vi "Get Pulse State.vi"(8 "error in (no error)":errorcluster, 11 "DAQmx Digitizer in":refnum<class "DAQmx Digitizer.lvclass">) -> (0 "error out":errorcluster, 1 "Result ready":bool, 2 "Armed":bool, 3 "DAQmx Digitizer out":refnum<class "DAQmx Digitizer.lvclass">, 4 "Recording compleste":bool)   [LabVIEW 2021, in "DAQmx Digitizer.lvclass"]
uses:
  DAQmx Digitizer.lvclass
  C:/GitHub/NHMFL_Core/Libraries/Instruments/Pulse Driver/Pulse Driver.lvclass
  Instruments/Pulse Driver/Pulse Driver.lvclass/Pulse Driver.ctl
  Instruments/Pulse Driver/Read Samples per read.vi
  Instruments/Pulse Driver/Read Samples per channel.vi
  Instruments/Pulse Driver/Read Current read position.vi
  DAQmx Digitizer.lvclass/DAQmx Digitizer.ctl
  <resource>/objmgr/daqmx.rc
panel:
  out "AvailSampPerChan 2":u32
  out "Samples per channel":i32
  out "Samples per read":i32=-1
  out "Current read position":i32
  out "AvailSampPerChan":u32
  out "RelativeTo":i32(ring)=10424 items=["First Sample"=10424, "Current Read Position"=10425, "Reference Trigger"=10426, "First Pretrigger Sample"=10427, "Most Recent Sample"=10428]
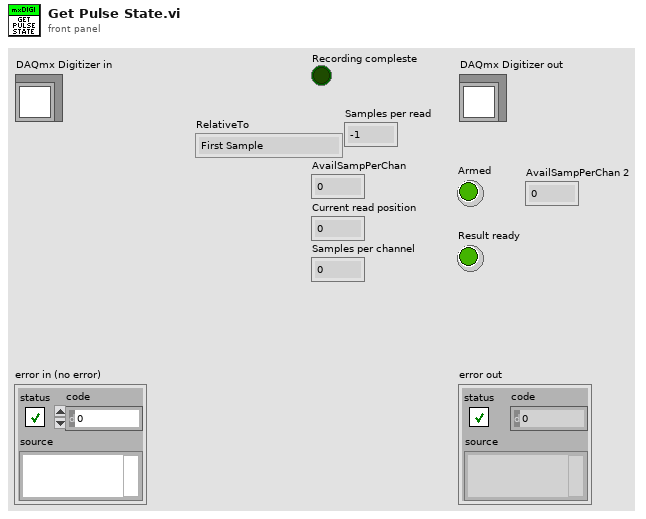
[diagram p1: front panel]
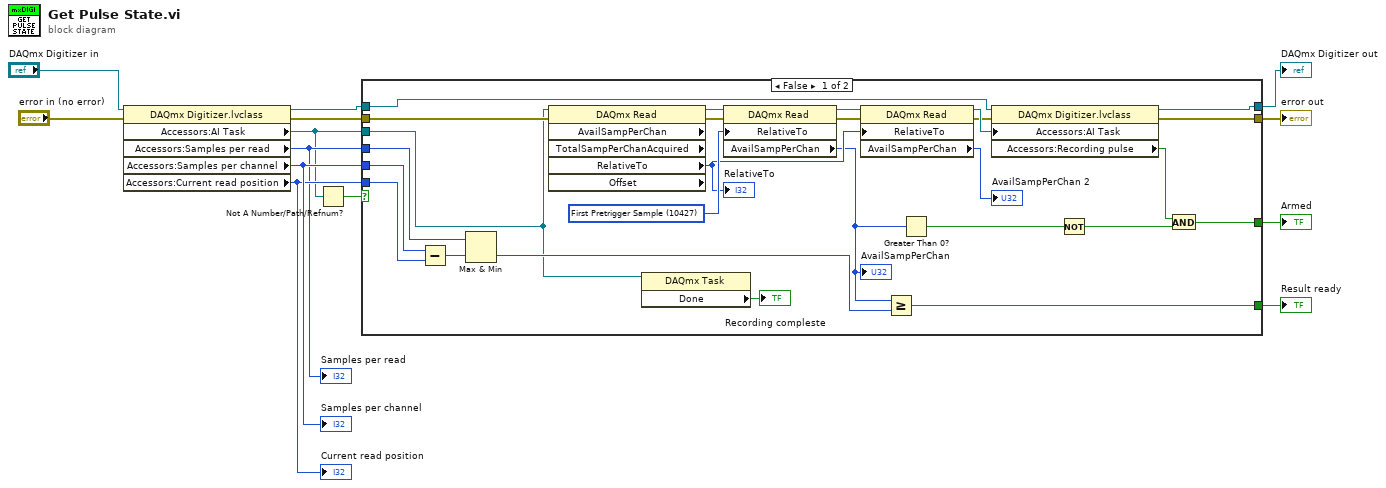
[diagram p0: block diagram]
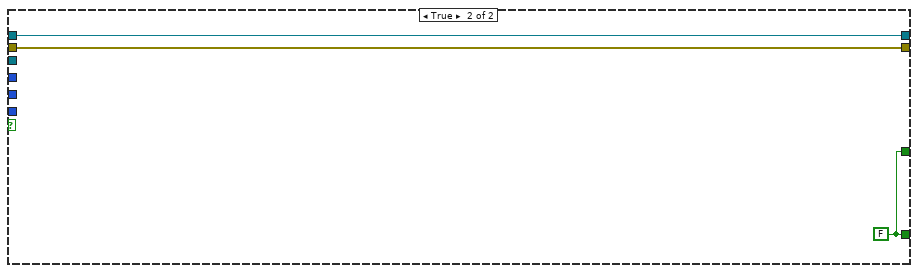
[diagram p2: hidden frame]
diagram:
  n1 = property class="DAQmx Digitizer.lvclass"(reference="DAQmx Digitizer in", error in="error in (no error)") -> (reference out=w11:refnum<class "DAQmx Digitizer.lvclass">, error out=w12:errorcluster, "Accessors:AI Task"=w2:refnum<k21>, "Accessors:Samples per read"=w5:i32, "Accessors:Samples per channel"=w13:i32, "Accessors:Current read position"=w6:i32)
  "Current read position" <- w6
  "Samples per read" <- w5
  "Samples per channel" <- w13
  n2 = Not A Number/Path/Refnum?(number/path/refnum=w2) -> (NaN/Path/Refnum?=w1:bool)
  n3 = case shown="False" w1 {
    tunnel: w13 -> [w39 _]
    tunnel: w12 -> [w37 w41]
    tunnel: w11 -> [w36 w40]
    tunnel: [w35 w42] -> w8
    tunnel: [w18 w42] -> w7
    tunnel: w6 -> [w33 _]
    tunnel: w5 -> [w31 _]
    tunnel: [w30 w41] -> w4
    tunnel: [w29 w40] -> w3
    tunnel: w2 -> [w15 _]
    frame False {
      w27 = 10427 items=["First Sample"=10424, "Current Read Position"=10425, "Reference Trigger"=10426, "First Pretrigger Sample"=10427, "Most Recent Sample"=10428] ("RelativeTo")
      n4 = Subtract(x=w39, y=w33) -> (x-y=w32:i32)
      n5 = Max & Min(x=w31, y=w32) -> (min(x,y)=w38:i32)  [unwired: 1 out]
      n6 = property class="DAQmx Read" props=["AvailSampPerChan", "TotalSampPerChanAcquired", "RelativeTo", "Offset"](reference=w15, error in=w37) -> (reference out=w28:refnum<k21>, error out=w21:errorcluster, "RelativeTo"=w25:i32)  [unwired: 3 out]
      "RelativeTo" <- w25
      n7 = property class="DAQmx Task"(reference=w15) -> ("Done"=→"Recording compleste":bool)  [unwired: 1 in, 2 out]
      n8 = property class="DAQmx Read"(reference=w28, error in=w21, "RelativeTo"=w27) -> (reference out=w26:refnum<k21>, error out=w22:errorcluster, "AvailSampPerChan"=w20:u32)
      "AvailSampPerChan" <- w20
      n9 = property class="DAQmx Read"(reference=w26, error in=w22, "RelativeTo"=w25) -> (reference out=w24:refnum<k21>, error out=w23:errorcluster, "AvailSampPerChan"=→"AvailSampPerChan 2":u32)
      n10 = Greater Or Equal?(x=w20, y=w38) -> (x >= y?=w35:bool)
      n11 = Greater Than 0?(x=w20) -> (x > 0?=w34:bool)
      n12 = property class="DAQmx Digitizer.lvclass"(reference=w36, error in=w23, "Accessors:AI Task"=w24) -> (reference out=w29:refnum<class "DAQmx Digitizer.lvclass">, error out=w30:errorcluster, "Accessors:Recording pulse"=w17:bool)
      n13 = Not(x=w34) -> (.not. x?=w19:bool)
      n14 = And(x=w17, y=w19) -> (x .and. y?=w18:bool)
    }
    frame True {
      w42 = FALSE
    }
  }
  "error out" <- w4
  "DAQmx Digitizer out" <- w3
  "Result ready" <- w8
  "Armed" <- w7
